vi "initHandler.vi"(8 "error in (no error)":errorcluster, 9 "Name":string, 10 "Level":T1(ring), 11 "Handler.UserEvent in":refnum<class "Handler.UserEvent.lvclass">) -> (0 "error out":errorcluster, 3 "Handler.UserEvent out":refnum<class "Handler.UserEvent.lvclass">)   [LabVIEW 2017, in "Error Log.lvlib" / "Handler.UserEvent.lvclass"]
uses:
  Handler.UserEvent.lvclass
  Handler/Handler.lvclass
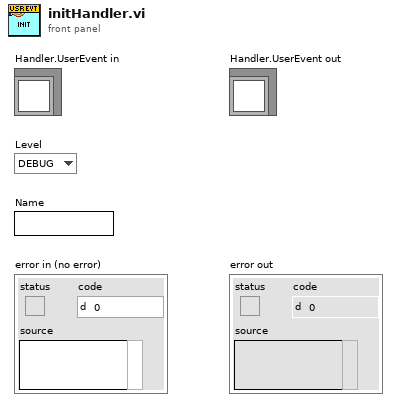
[diagram p1: front panel]
types:
  T1 = enum16{"DEBUG", "INFO", "WARNING", "ERROR", "CRITICAL"}
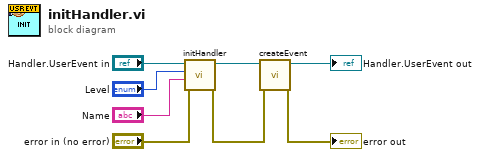
[diagram p0: block diagram]
diagram:
  n1 = call-parent "initHandler.vi"("error in (no error)"="error in (no error)", "Name"="Name", "Level"="Level", "Handler in"="Handler.UserEvent in") -> ("error out"=w2:errorcluster, "Handler out"=w4:refnum<class "Handler.UserEvent.lvclass">)  [unwired: 6 in]
  n2 = call-dynamic "createEvent.vi"("error in (no error)"=w2, "Handler.UserEvent in"=w4) -> ("error out"=→"error out":errorcluster, "Handler.UserEvent out"=→"Handler.UserEvent out":refnum<class "Handler.UserEvent.lvclass">)  [unwired: 8 in]
